vi "GenerateTagPeriod.vi"(8 "Error in":errorcluster, 9 "TaggingPeriod (pws)":i32, 10 "TagMarkerDuration (pws)":i32, 11 "Tag num":u32) -> (0 "Error Out":errorcluster, 2 "TagDataLength (pws)":i32, 3 "TagPeriodData":digitalwaveform(waveform)={"t0"=timestamp(0 s since 1904-01-01), "dt"=0.0, "Y"={"transitions"=[], "data"=[]}, "error"={"status"=FALSE, "code"=37421928, "source"=""}})   [LabVIEW 2017]
uses:
  <vilib>/Waveform/DWDTOps.llb/DWDT Digital Size.vi
  <vilib>/Waveform/DWDTOps.llb/DWDT Append Digital Samples.vi
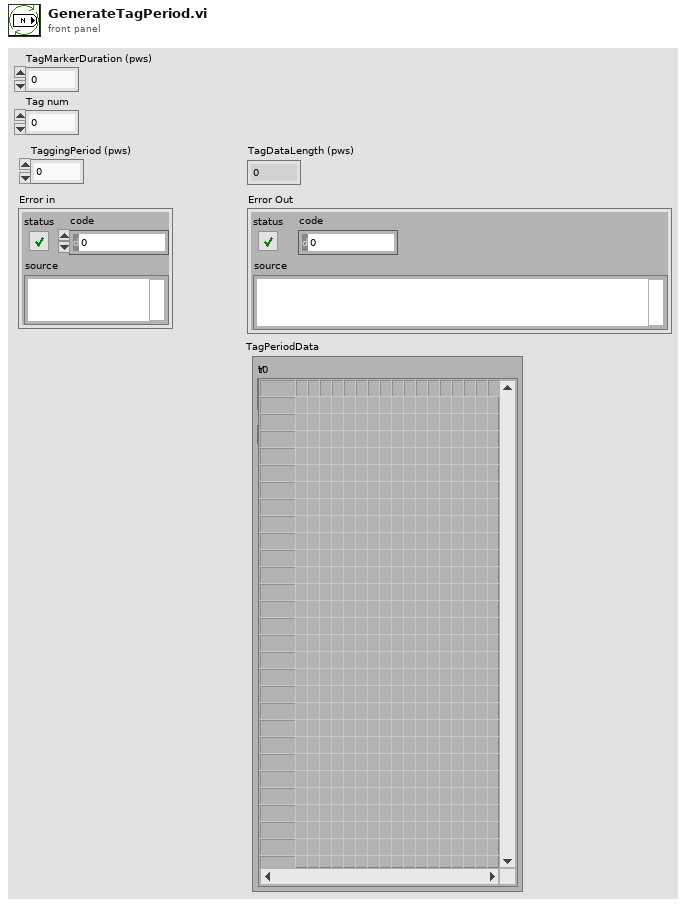
[diagram p1: front panel]
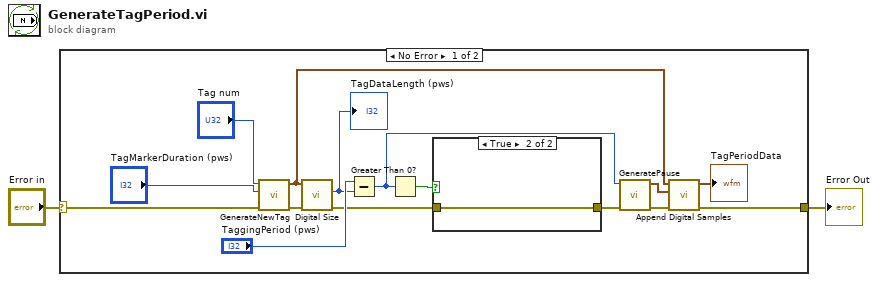
[diagram p0: block diagram]
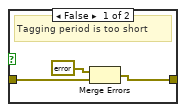
[diagram p2: hidden frame]
diagram:
  n1 = case shown="No Error" "Error in" {
    selector: "Error in" -> [w15 w22]
    tunnel: [w14 w22] -> w1
    frame No Error {
      n2 = call "GenerateNewTag.vi"("Error in"=w15, "TagMarkerDuration (pws)"="TagMarkerDuration (pws)", "Tag num"="Tag num") -> ("Error Out"=w8:errorcluster, "digital waveform"=w11:digitalwaveform)  [unwired: 7 in]
      n3 = call-poly <vilib>:"Digital Size.vi"("error in (no error)"=w8, "digital waveform in"=w11) -> ("error out"=w4:errorcluster, "number of samples"=w9:i32)  [unwired: 6 in, 2 out]
      "TagDataLength (pws)" <- w9
      n4 = Subtract(x="TaggingPeriod (pws)", y=w9) -> (x-y=w6:i32)
      n5 = Greater Than 0?(x=w6) -> (x > 0?=w5:bool)
      n6 = case shown="True" w5 {
        tunnel: w4 -> [w19 w21]
        tunnel: [w18 w21] -> w3
        frame False {
          # "Tagging period is too short"
          n7 = Merge Errors(errorcluster {"status"=TRUE, "code"=-1967345148, "source"="Warning! Tag data does not fit in period. \nPlease increase tag period and restart VI."} ("error in (no error)"), w19) -> (w18:errorcluster)
        }
        frame True {
        }
      }
      n8 = call "GeneratePause.vi"("Error in"=w3, "PauseDuration (pws)"=w6) -> ("Error Out"=w13:errorcluster, "digital waveform"=w12:digitalwaveform)  [unwired: 8 in]
      n9 = call-poly <vilib>:"Append Digital Samples.vi"("error in (no error)"=w13, "digital waveform B"=w12, "digital waveform A"=w11) -> ("error out"=w14:errorcluster, "digital waveform out"=→"TagPeriodData":digitalwaveform)  [unwired: 7 in]
    }
    frame Error {
    }
  }
  "Error Out" <- w1
